vi "Login SignUp.vi"() -> ()   [LabVIEW 2022 SP3]
panel:
  out "Tab Control":enum32{"Login", "SignUp", "YouAreOnline"}(tab)
  in  "Pasword":string
  in  "Nickname":string
  in  "LogIn":bool
  in  "stop":bool
  in  "GotoSignUpPage":bool
  in  "SignUp":bool
  in  "Enter your pasword":string
  in  "Enter your nickname":string
  in  "GoToLogInPage":bool
  in  "stop 2":bool
  out "concatenated string":string
  out "You are online":bool
  in  "stop 3":bool
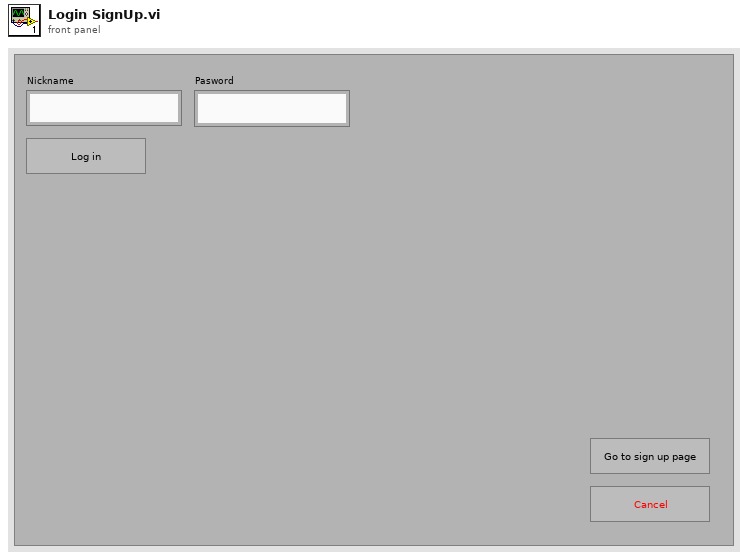
[diagram p1: front panel]
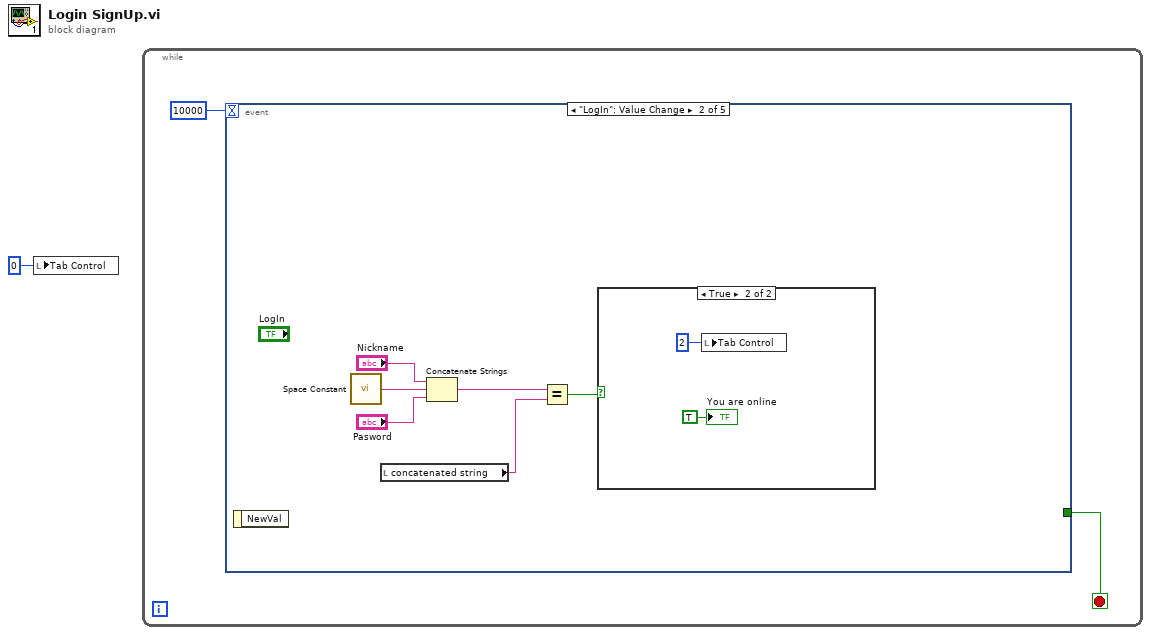
[diagram p0: block diagram]
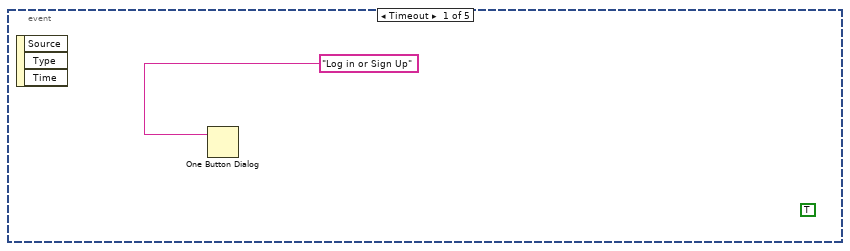
[diagram p2: hidden frame]
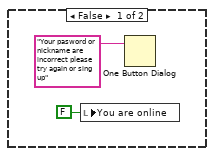
[diagram p3: hidden frame]
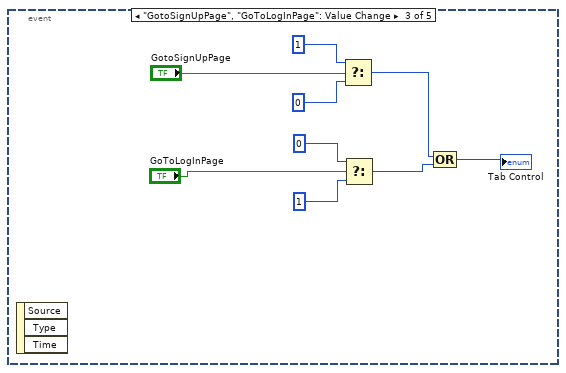
[diagram p4: hidden frame]
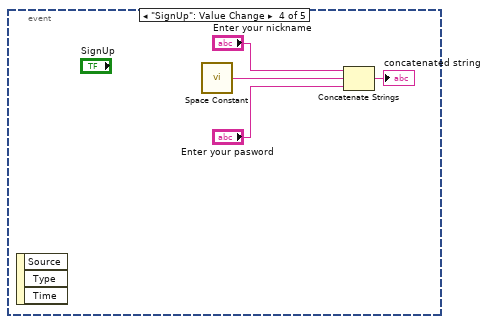
[diagram p5: hidden frame]
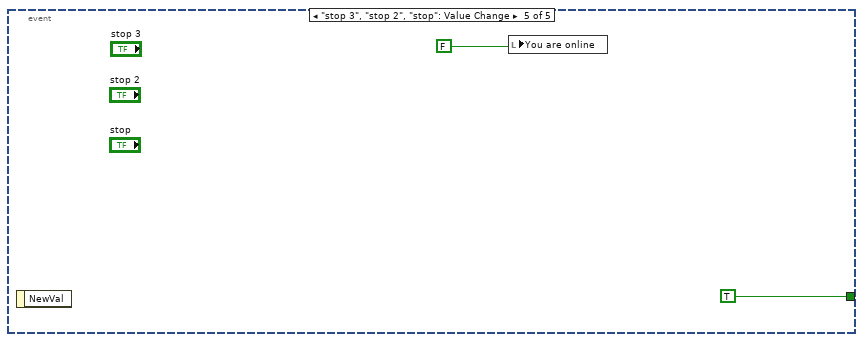
[diagram p6: hidden frame]
diagram:
  n1 = local write "Tab Control"(0 ("Tab Control")) -> ()
  n2 = while {
    stop <- w2 stop-if-true
    n3 = event shown="[1] \"LogIn\": Value Change" {
      selector: _ -> [_ _ _ _ _]
      dyn-events: _ -> [_ _ _ _ _]
      timeout: 10000 -> [_ _ _ _ _]
      tunnel: [_ _ _ _ TRUE] -> w2
      event Timeout {
        (unwired) TRUE
        n4 = event-data() -> ()  [unwired: 1 in, 3 out]
        n5 = One Button Dialog(message="Log in or Sign Up") -> ()  [unwired: 1 in, 1 out]
      }
      event "LogIn": Value Change {
        n6 = event-data() -> ()  [unwired: 1 in, 1 out]
        n7 = call <vilib>:"Space Constant.vi"() -> ("String"=w10:string)
        n8 = local read "concatenated string"() -> (w5:string)
        n9 = Concatenate Strings("Nickname", w10, "Pasword") -> (w7:string)
        n10 = Equal?(x=w7, y=w5) -> (x = y?=w6:bool)
        n11 = case shown="True" w6 {
          frame False {
            n12 = local write "You are online"(FALSE ("You are online")) -> ()
            n13 = One Button Dialog(message="Your pasword or nickname are incorrect please try again or sing up") -> ()  [unwired: 1 in, 1 out]
          }
          frame True {
            n14 = local write "Tab Control"(2 ("Tab Control")) -> ()
            "You are online" <- TRUE ("Boolean")
          }
        }
      }
      event "GotoSignUpPage", "GoToLogInPage": Value Change {
        n15 = event-data() -> ()  [unwired: 1 in, 3 out]
        n16 = Select(t=1, s="GotoSignUpPage", f=0) -> (s? t:f=w16:i32)
        n17 = Select(t=0, s="GoToLogInPage", f=1) -> (s? t:f=w17:i32)
        n18 = Compound Arithmetic op=OR(w16, w17) -> (→"Tab Control":i32)
      }
      event "SignUp": Value Change {
        n19 = event-data() -> ()  [unwired: 1 in, 3 out]
        n20 = call <vilib>:"Space Constant.vi"() -> ("String"=w25:string)
        n21 = Concatenate Strings("Enter your nickname", w25, "Enter your pasword") -> (→"concatenated string":string)
      }
      event "stop 3", "stop 2", "stop": Value Change {
        n22 = event-data() -> ()  [unwired: 1 in, 1 out]
        n23 = local write "You are online"(FALSE) -> ()
      }
    }
  }
